vi "Time2Points.vi"(1 "Time [ms]":dbl, 3 "Sample Rate":dbl) -> (0 "Points":i32)   [LabVIEW 2016]
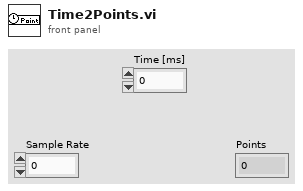
[diagram p1: front panel]
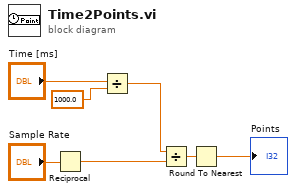
[diagram p0: block diagram]
diagram:
  n1 = Reciprocal(x="Sample Rate") -> (1/x=w6:dbl)
  n2 = Divide(x="Time [ms]", y=1000.0) -> (x/y=w3:dbl)
  n3 = Divide(x=w3, y=w6) -> (x/y=w2:dbl)
  n4 = Round To Nearest(number=w2) -> (nearest integer value=→"Points":dbl)
